vi "test Import Different Module.vi"(8 "error in (no error)":errorcluster, 11 "TestCase in":refnum<class "SLSC Switch Import Export Unit Tests.lvclass">) -> (0 "error out":errorcluster, 3 "TestCase out":refnum<class "SLSC Switch Import Export Unit Tests.lvclass">)   [LabVIEW 2020, in "SLSC Switch Import Export Unit Tests.lvclass"]
uses:
  SLSC Switch Import Export Unit Tests.lvclass
  Shared/Endpoint Configuration Cluster.ctl
  Shared/Endpoint Configuration Enum.ctl
  SLSC Switch Import Export Unit Tests.lvclass/SLSC Switch Import Export Unit Tests.ctl
  <vilib>/NI VeriStand/Custom Device API/Get Item Property (U32).vi
  <vilib>/addons/_JKI Toolkits/VI Tester/TestCase.llb/TestCase.lvclass
  <vilib>/NI/NI VeriStand Custom Device Import and Export Tool/ImportExport.lvlib
  Scripting/SLSC Switch Scripting.lvlib
  Shared/VeriStand System Definition Test Utilities/VeriStand System Definition Test Utilities.lvlib
  Shared/SLSC Switch Shared.lvlib
  <vilib>/NI VeriStand/Custom Device API/Custom Device API.lvlib
  C:/Program Files (x86)/National Instruments/LabVIEW 2020/vi.lib/addons/_JKI Toolkits/VI Tester/TestCase.llb/TestCase.lvclass
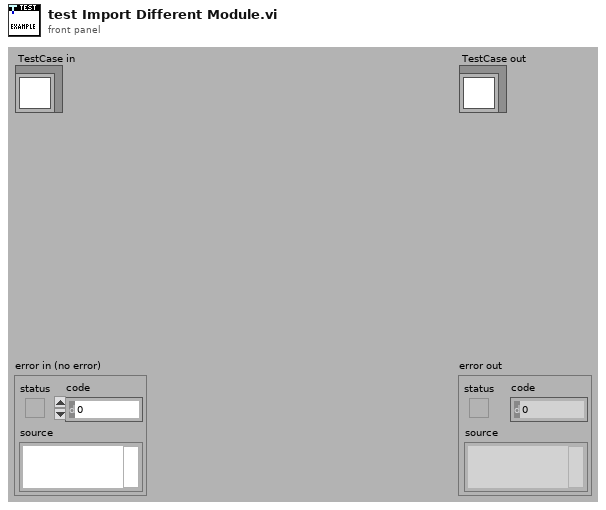
[diagram p1: front panel]
types:
  T1 = typedef "SLSC Switch Shared.lvlib/Endpoint Configuration Cluster.ctl" = cluster{"Endpoint":string, "Configuration":T2}
  T2 = typedef "SLSC Switch Shared.lvlib/Endpoint Configuration Enum.ctl" = enum16{"Load", "Source", "Configuration"}
  T3 = cluster{"Ignore Properties":string[], "Ignore Top Level Name":bool}
  T4 = typedef "Custom Device API.lvlib/Custom Device Item Ref.ctl" = u64
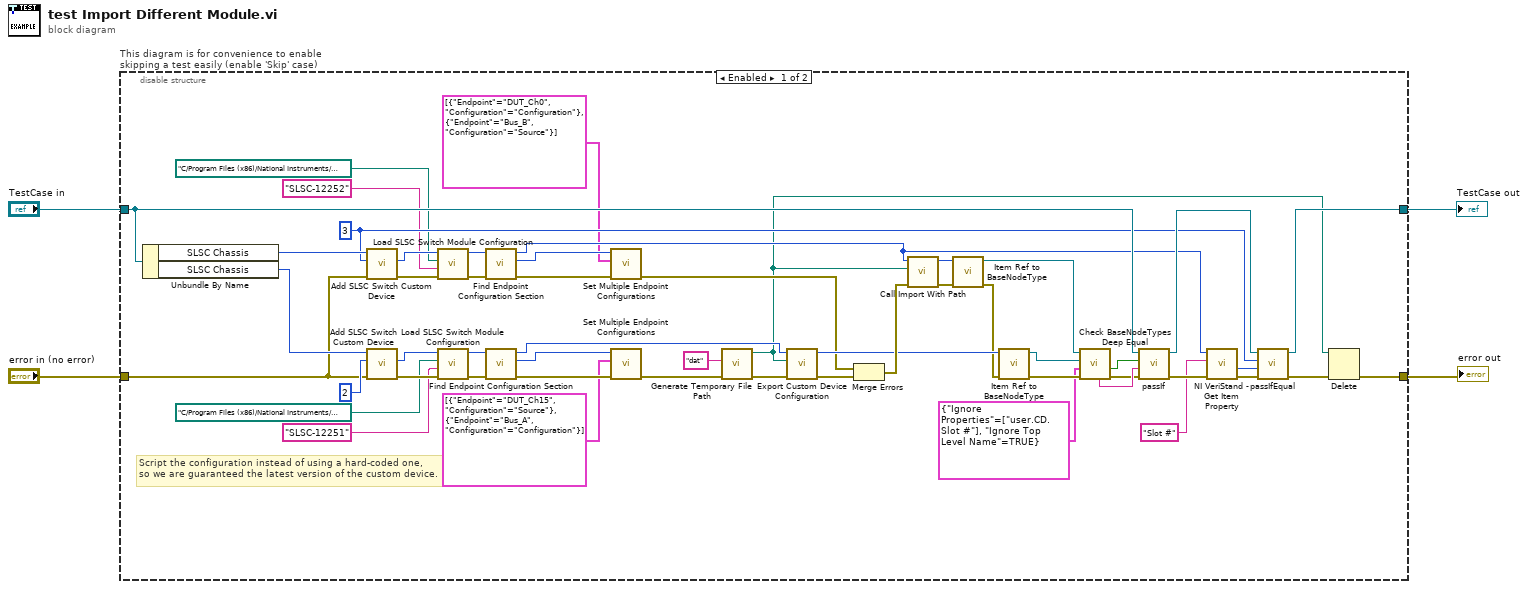
[diagram p0: block diagram]
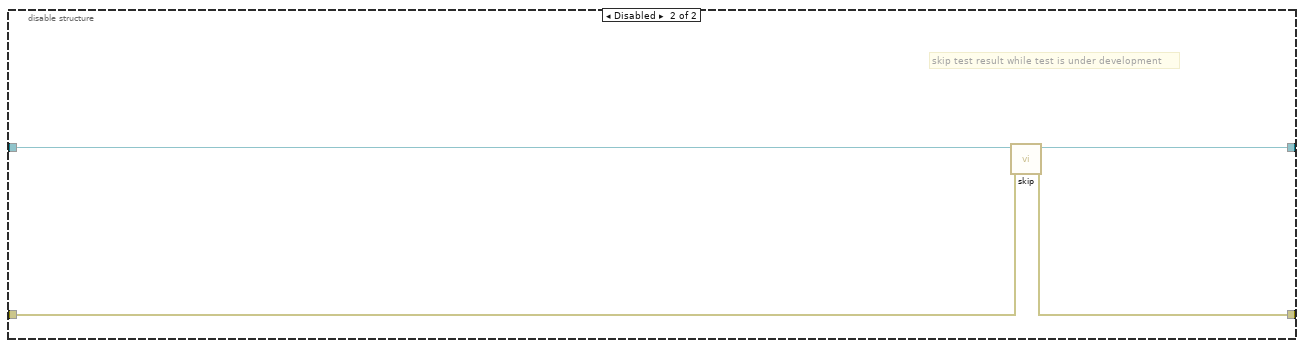
[diagram p2: hidden frame]
diagram:
  n1 = disable-structure "This diagram is for convenience to enable skipping a test easily (enable 'Skip' case)" shown="Enabled" {
    disable-tunnel: "TestCase in" -> [w43 w60]
    disable-tunnel: [w25 w58] -> w1
    disable-tunnel: [w6 w59] -> w3
    disable-tunnel: "error in (no error)" -> [w37 w57]
    frame Enabled {
      w22 = u32 3 ("slot number")
      # "Script the configuration instead of using a hard-coded one,\nso we are guaranteed the latest version of the custom device."
      n2 = Unbundle By Name(w43) -> ("SLSC Chassis"=w38:u64, "SLSC Chassis"=w56:u64)
      n3 = call "Add SLSC Switch Custom Device.vi"("error in"=w37, "slot number"=w22, "slsc chassis in"=w38) -> ("error out"=w19:errorcluster, "slsc switch custom device"=w15:T4)  [unwired: 6 in, 1 out]
      n4 = call "Add SLSC Switch Custom Device.vi"("error in"=w37, "slot number"=u32 2, "slsc chassis in"=w56) -> ("error out"=w36:errorcluster, "slsc switch custom device"=w34:T4)  [unwired: 6 in, 1 out]
      n5 = call "Load SLSC Switch Module Configuration.vi"("error in"=w19, "product name"="SLSC-12252", "switches json file"=path "C:/Program Files (x86)/National Instruments/Shared/NI-SLSC Switch/Modules/SLSC-12252-switches.json", "slsc switch custom device in"=w15) -> ("error out"=w18:errorcluster, "slsc switch custom device out"=w20:T4)  [unwired: 6 in]
      n6 = call "Load SLSC Switch Module Configuration.vi"("error in"=w36, "product name"="SLSC-12251", "switches json file"=path "C:/Program Files (x86)/National Instruments/Shared/NI-SLSC Switch/Modules/SLSC-12251-switches.json", "slsc switch custom device in"=w34) -> ("error out"=w35:errorcluster, "slsc switch custom device out"=w32:T4)  [unwired: 6 in]
      n7 = call "Find Endpoint Configuration Section.vi"("error in"=w18, "slsc switch custom device in"=w20) -> ("error out"=w14:errorcluster, "endpoint configuration"=w12:T4, "slsc switch custom device out"=w11:T4)  [unwired: 7 in]
      n8 = call "Find Endpoint Configuration Section.vi"("error in"=w35, "slsc switch custom device in"=w32) -> ("error out"=w33:errorcluster, "endpoint configuration"=w30:T4, "slsc switch custom device out"=w29:T4)  [unwired: 7 in]
      n9 = call "Set Multiple Endpoint Configurations.vi"("error in"=w14, "endpoint configurations"=T1[] [{"Endpoint"="DUT_Ch0", "Configuration"=enum."Configuration"}, {"Endpoint"="Bus_B", "Configuration"=enum."Source"}], "endpoint configuration in"=w12) -> ("error out"=w10:errorcluster)  [unwired: 7 in, 1 out]
      n10 = call "Set Multiple Endpoint Configurations.vi"("error in"=w33, "endpoint configurations"=T1[] [{"Endpoint"="DUT_Ch15", "Configuration"=enum."Source"}, {"Endpoint"="Bus_A", "Configuration"=enum."Configuration"}], "endpoint configuration in"=w30) -> ("error out"=w31:errorcluster)  [unwired: 7 in, 1 out]
      n11 = call <vilib>:"Generate Temporary File Path.vi"("error in (no error)"=w31, "Temporary File Extension (tmp)"="dat") -> ("error out"=w53:errorcluster, "Unique Temporary File Path"=w5:path)  [unwired: 8 in]
      n12 = call <vilib>:"Export Custom Device Configuration.vi"("error in (no error)"=w53, "Path"=w5, "ID"=w29) -> ("error out"=w52:errorcluster, "ID out"=w49:u64)  [unwired: 7 in]
      n13 = Merge Errors(w10, w52) -> (w51:errorcluster)
      n14 = call "Call Import With Path.vi"("error in (no error)"=w51, "Path"=w5, "Node Ptr"=w11) -> ("error out"=w48:errorcluster, "Node Ptr out"=w50:u64)  [unwired: 7 in]
      n15 = call "Item Ref to BaseNodeType.vi"("error in (no error)"=w48, "Item Ref"=w50) -> ("error out"=w47:errorcluster, "BaseNodeType"=w40:refnum<k24>)  [unwired: 8 in]
      n16 = call "Item Ref to BaseNodeType.vi"("error in (no error)"=w47, "Item Ref"=w49) -> ("error out"=w46:errorcluster, "BaseNodeType"=w45:refnum<k24>)  [unwired: 8 in]
      n17 = call "Check BaseNodeTypes Deep Equal.vi"("error in (no error)"=w46, "Settings"=T3 {"Ignore Properties"=["user.CD.Slot #"], "Ignore Top Level Name"=TRUE}, "BaseNodeType 2"=w45, "BaseNodeType 1"=w40) -> ("error out"=w39:errorcluster, "Equal?"=w42:bool, "Inequality context"=w41:string)  [unwired: 3 in, 2 out]
      n18 = call-dynamic "passIf.vi"("error in (no error)"=w39, "message (\"\")"=w41, "pass"=w42, "TestCase in"=w43) -> ("error out"=w44:errorcluster, "TestCase out"=w26:refnum<class "SLSC Switch Import Export Unit Tests.lvclass">)  [unwired: 6 in]
      n19 = call-poly <vilib>:"NI VeriStand - Get Item Property.vi"("error in (no error)"=w44, "Property Name"="Slot #", "Item Ref in"=w11) -> ("error out"=w24:errorcluster, "Value"=w23:u32)  [unwired: 5 in, 2 out]
      n20 = call-dynamic "passIfEqual.vi"("error in (no error)"=w24, "y"=w23, "x"=w22, "TestCase in"=w26) -> ("error out"=w27:errorcluster, "TestCase out"=w25:refnum<class "SLSC Switch Import Export Unit Tests.lvclass">)  [unwired: 6 in]
      n21 = Delete(path (use dialog)=w5, error in=w27) -> (error out=w6:errorcluster)  [unwired: 3 in, 2 out]
    }
    frame Disabled {
      # "skip test result while test is under development"
      n22 = call <vilib>:"skip.vi"("error in (no error)"=w57, "TestCase in"=w60) -> ("error out"=w59:errorcluster, "TestCase out"=w58:refnum<class "SLSC Switch Import Export Unit Tests.lvclass">)  [unwired: 8 in]
    }
  }
  "error out" <- w3
  "TestCase out" <- w1
